vi "View_Log.vi"() -> ()   [LabVIEW 2011]
doc: "This VI functions as a new window in which the user can view, save, or clear the global log text."
uses:
  low_level_proc/globals.vi
panel:
  in  "Clear Log":bool
  in  "Close":bool
  in  "Save Log":bool
  out "Log":string
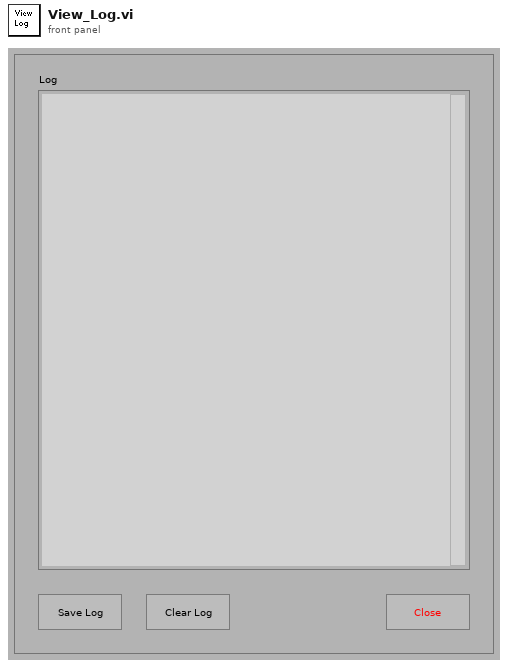
[diagram p1: front panel]
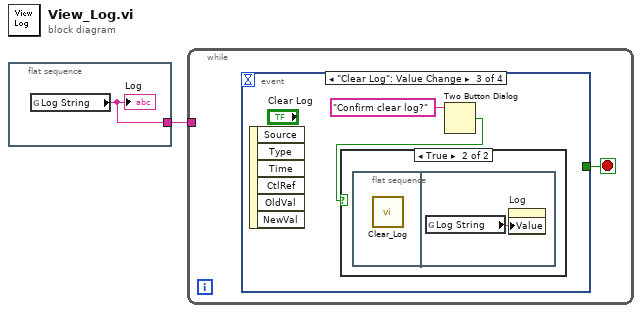
[diagram p0: block diagram]
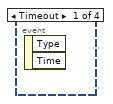
[diagram p2: hidden frame]
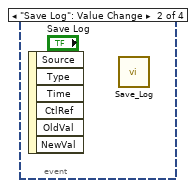
[diagram p3: hidden frame]
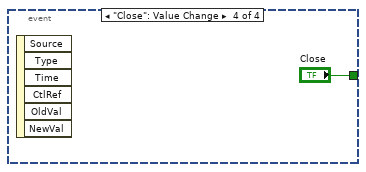
[diagram p5: hidden frame]
diagram:
  n1 = flat-sequence {
    tunnel: [w2] -> w1
    frame #0 {
      n2 = global read "globals.vi" "Log String"() -> (w2:string)
      "Log" <- w2
    }
  }
  n3 = while {
    tunnel: w1 -> [_]
    stop <- w3 stop-if-true
    n4 = event shown="[2] \"Clear Log\": Value Change" {
      selector: _ -> [_ _ _ _]
      dyn-events: _ -> [_ _ _ _]
      timeout: _ -> [_ _ _ _]
      tunnel: [_ _ _ "Close"] -> w3
      event Timeout {
        n5 = event-data() -> ()  [unwired: 3 out]
      }
      event "Save Log": Value Change {
        n6 = event-data() -> ()  [unwired: 7 out]
        n7 = call "Save_Log.vi"() -> ()  [unwired: 2 out]
      }
      event "Clear Log": Value Change {
        n8 = event-data() -> ()  [unwired: 7 out]
        n9 = Two Button Dialog(message="Confirm clear log?") -> (T button?=w4:bool)  [unwired: 2 in]
        n10 = case shown="True" w4 {
          frame False {
          }
          frame True {
            n11 = flat-sequence {
              frame #0 {
                n12 = call "Clear_Log.vi"() -> ()  [unwired: 12 out]
              }
              frame #1 {
                n13 = global read "globals.vi" "Log String"() -> (w6:string)
                n14 = property on="Log" class="Str"("Value"=w6) -> ()  [unwired: 2 in, 2 out]
              }
            }
          }
        }
      }
      event "Close": Value Change {
        n15 = event-data() -> ()  [unwired: 7 out]
      }
    }
  }
